vi "Init Spawn.vi"(10 "Spawn":T1) -> (3 "Base Spawn out":refnum<class "Base Spawn.lvclass">)   [LabVIEW 2025, in "jettl.lvlib" / "Spawn.lvlib" / "Base Spawn.lvclass"]
uses:
  Base Spawn.lvclass
  Spawn.ctl
  Attributes/Attributes/Attributes.lvclass
  Actor/Actor.lvclass
  Base Spawn.lvclass/Base Spawn.ctl
  jettl.lvlib
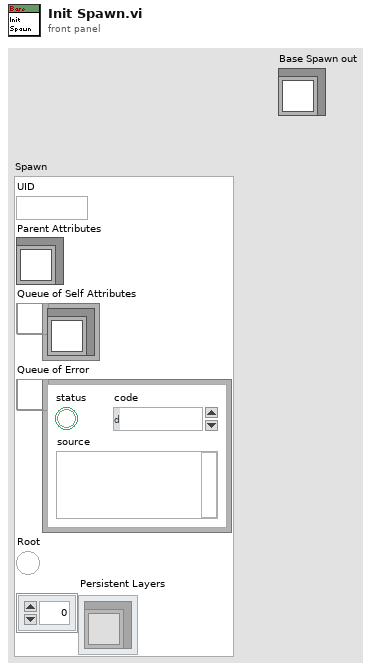
[diagram p1: front panel]
types:
  T1 = typedef "jettl.lvlib/Spawn.ctl" = cluster{"UID":string, "Parent Attributes":refnum<class "Attributes.lvclass">, "Queue of Self Attributes":refnum<queue>, "Queue of Error":refnum<queue>, "Root":bool, "Persistent Layers":refnum<class "Actor.lvclass">[]}
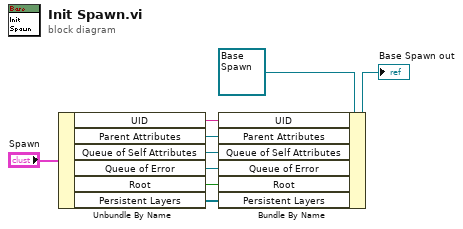
[diagram p0: block diagram]
diagram:
  n1 = Unbundle By Name("Spawn") -> ("UID"=w6:string, "Parent Attributes"=w5:refnum<class "Attributes.lvclass">, "Queue of Self Attributes"=w4:refnum<queue>, "Queue of Error"=w3:refnum<queue>, "Root"=w2:bool, "Persistent Layers"=w1:refnum<class "Actor.lvclass">[])
  n2 = Bundle By Name(cluster=refnum<class "Base Spawn.lvclass"> refnum ("Base Spawn out"), "UID"=w6, "Parent Attributes"=w5, "Queue of Self Attributes"=w4, "Queue of Error"=w3, "Root"=w2, "Persistent Layers"=w1) -> (→"Base Spawn out":refnum<class "Base Spawn.lvclass">)
